vi "code1.vi"() -> ()   [LabVIEW 2019]
panel:
  out "Waveform Chart":u8(graph)
  in  "Horizontal Pointer Slide":u8(slide) scale=0.0..10.0
  out "Output String":string
  in  "Input String":string
  out "Tank":dbl(slide) scale=0.0..1000.0
  in  "B":dbl
  in  "A":dbl
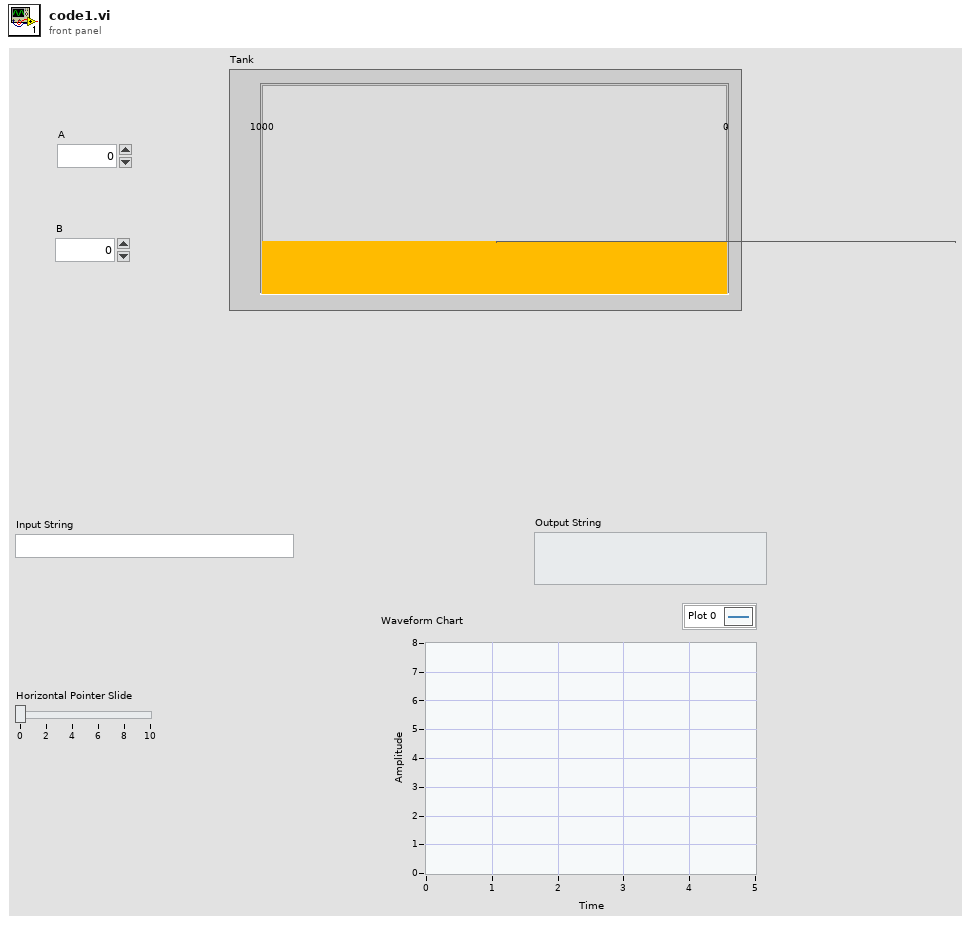
[diagram p1: front panel]
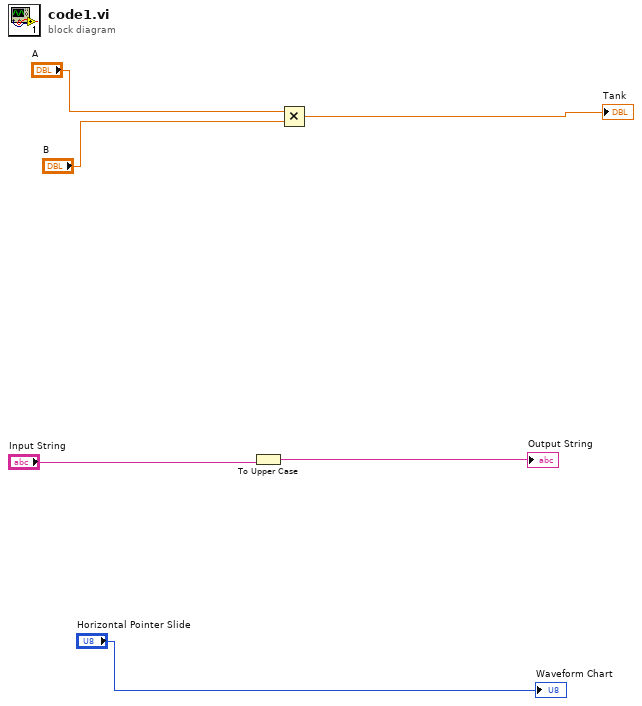
[diagram p0: block diagram]
diagram:
  n1 = To Upper Case(1:"Input String") -> (0:→"Output String":string)
  n2 = Multiply(x="A", y="B") -> (x*y=→"Tank":dbl)
  "Waveform Chart" <- "Horizontal Pointer Slide"
